vi "Random Number In Range.vi"(1 "하위 리미트":u32, 2 "상위 리미트":u32=1) -> (0 "임의의 수":u32)   [LabVIEW 2010]
doc: "상위 리미트와 하위 리미트로 지정된 범위안에서 임의의 수를 반환합니다."
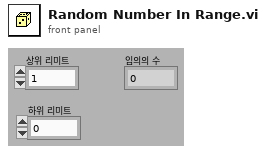
[diagram p1: front panel]
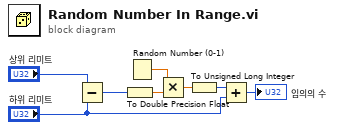
[diagram p0: block diagram]
diagram:
  n1 = Subtract(x="상위 리미트", y="하위 리미트") -> (x-y=w6:u32)
  n2 = To Double Precision Float(number=w6) -> (double precision float=w2:dbl)
  n3 = Random Number (0-1)() -> (number: 0 to 1=w3:dbl)
  n4 = Multiply(x=w3, y=w2) -> (x*y=w8:dbl)
  n5 = To Unsigned Long Integer(number=w8) -> (unsigned 32bit integer=w1:u32)
  n6 = Add(x=w1, y="하위 리미트") -> (x+y=→"임의의 수":u32)
